vi "ArmFF_MinAchieveVelocity.vi"(8 "Acceleration":dbl, 9 "Angle":dbl, 10 "MaxVoltage":dbl, 11 "in ARM_FF":T1 {"kCos" format="%13.5p"; "Ka" format="%13.5p"; "Kv" format="%13.5p"; "Ks" format="%13.5p"}) -> (3 "MinVelocity":dbl)   [LabVIEW 2019, in "Trajectory_Library.lvlib"]
doc: "Calculates the minimum achievable velocity given a maximum voltage supply, a position, and an acceleration. Useful for ensuring that velocity and acceleration constraints for a trapezoidal profile are simultaneously achievable - enter the acceleration constraint, and this will give you a simultaneously-achievable velocity constraint.\n \nInputs: \n - ArmFF -- The ArmFF data cluster\n - maxVoltage -- The maximum voltage that can be supplied to the arm.\n - angle -- The angle of the arm.\n - acceleration -- The acceleration of the arm.\n\nOutputs:\n - MinVelocity -- The minimum possible velocity at the given acceleration and angle."
uses:
  Trajectory_Library.lvlib
  TypeDef/ARM_FF.ctl
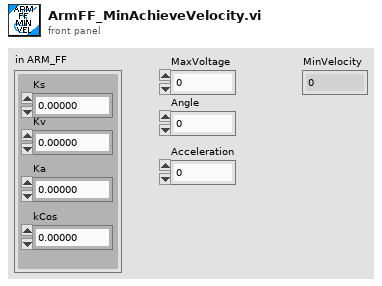
[diagram p1: front panel]
types:
  T1 = typedef "Trajectory_Library.lvlib/ARM_FF.ctl" = cluster{"Ks":dbl, "Kv":dbl, "Ka":dbl, "kCos":dbl}
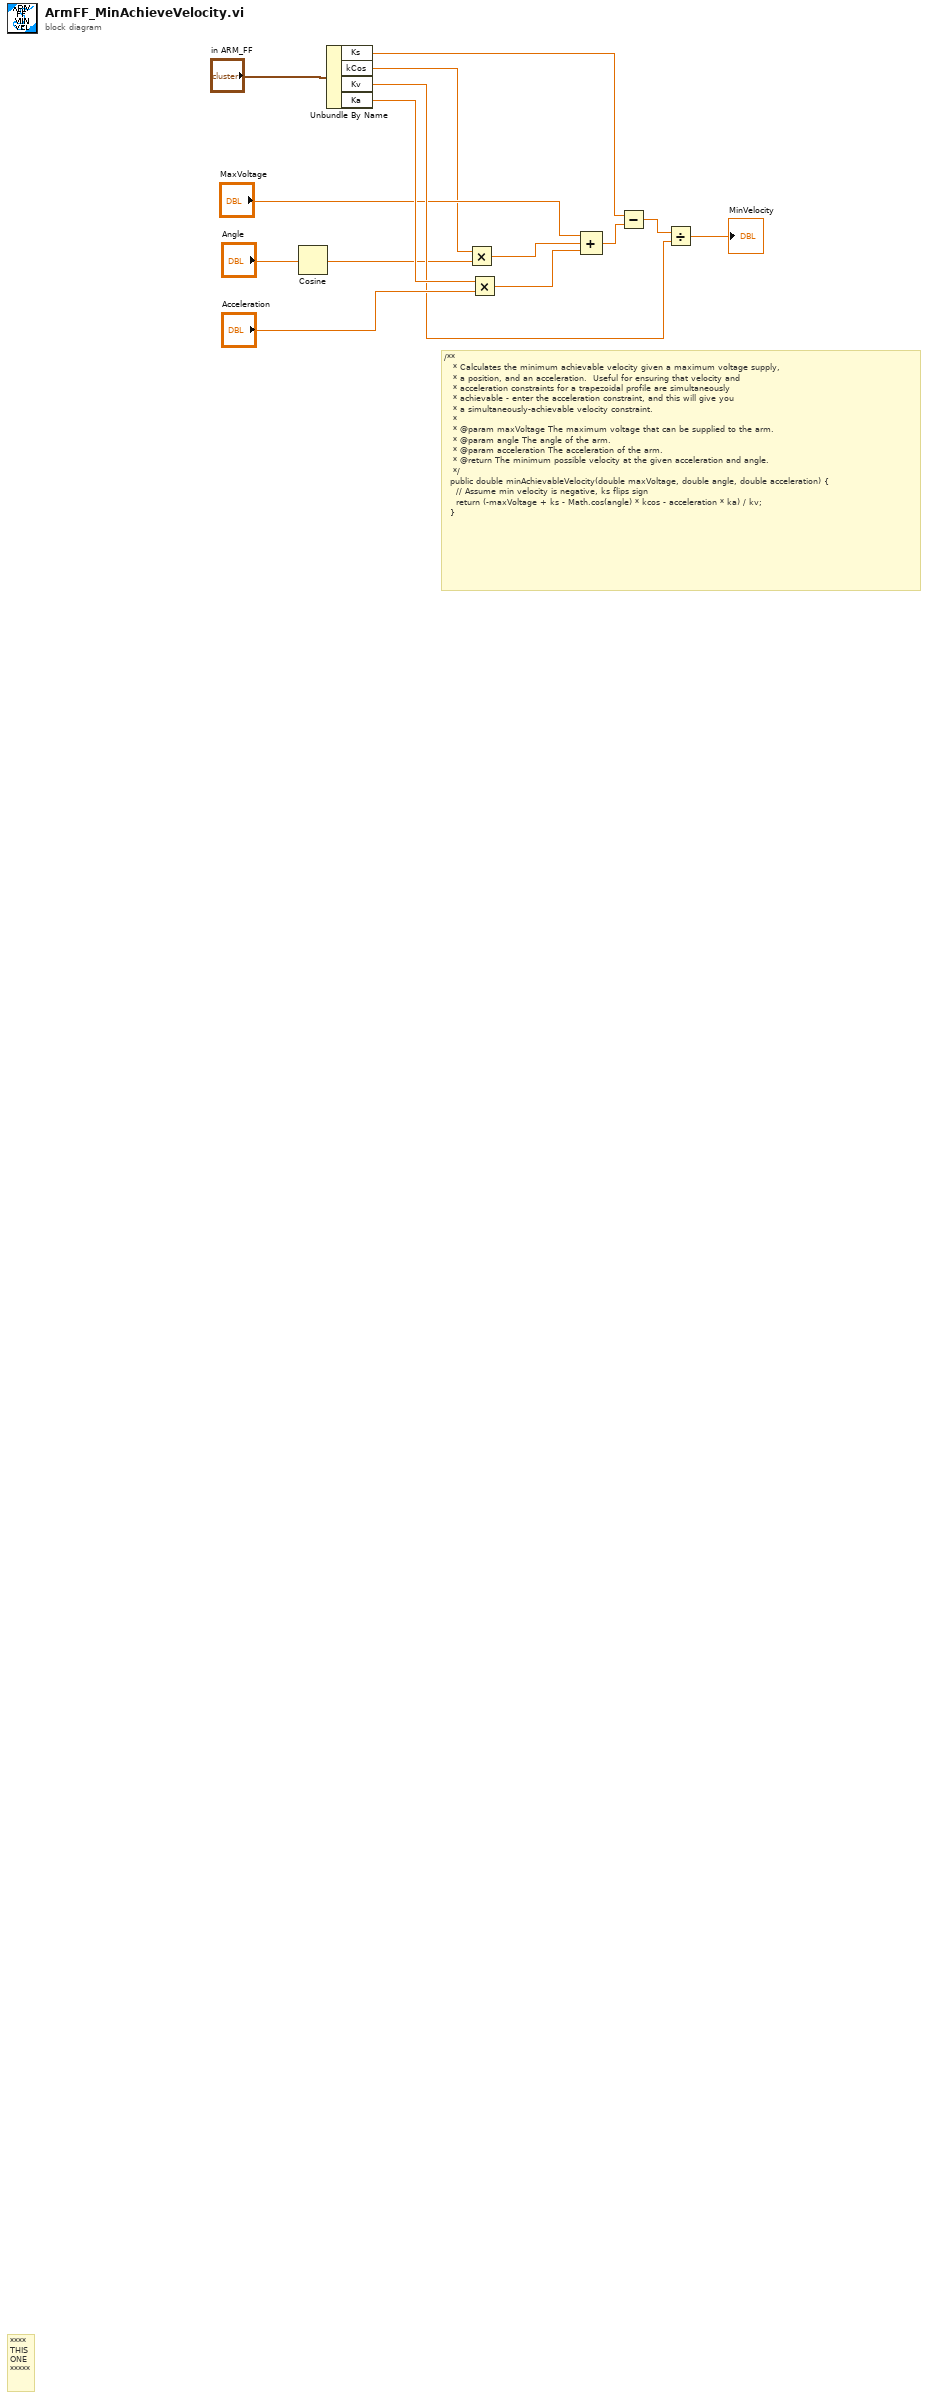
[diagram p0: block diagram]
diagram:
  # "/**\n   * Calculates the minimum achievable velocity given a maximum voltage supply,\n   * a position, and an acceleration.  Useful for ensuring that velocity and\n   * acceleration constraints for a trapezoidal profile are simultaneously\n   * achievable - enter the acceleration constraint, and this will give you\n   * a simultaneously-achievable velocity constraint.\n   *\n   * @param maxVoltage The maximum voltage that can be supplied to the arm.\n   * @param angle The angle of the arm.\n   * @param acceleration The acceleration of the arm.\n   * @return The minimum possible velocity at the given acceleration and angle.\n   */\n  public double minAchievableVelocity(double maxVoltage, double angle, double acceleration) {\n    // Assume min velocity is negative, ks flips sign\n    return (-maxVoltage + ks - Math.cos(angle) * kcos - acceleration * ka) / kv;\n  }"
  # "****\nTHIS\nONE\n*****"
  n1 = Cosine(x="Angle") -> (cos(x)=w2:dbl)
  n2 = Unbundle By Name("in ARM_FF") -> ("Ks"=w6:dbl, "kCos"=w1:dbl, "Kv"=w8:dbl, "Ka"=w11:dbl)
  n3 = Multiply(x=w1, y=w2) -> (x*y=w13:dbl)
  n4 = Multiply(x=w11, y="Acceleration") -> (x*y=w12:dbl)
  n5 = Compound Arithmetic op=ADD("MaxVoltage", w13, w12) -> (w5:dbl)
  n6 = Subtract(x=w6, y=w5) -> (x-y=w7:dbl)
  n7 = Divide(x=w7, y=w8) -> (x/y=→"MinVelocity":dbl)
